vi "Config Reference Point.vi"(8 "error in":errorcluster, 9 "Loss (0 jpF)":dbl min=-99999999.0 max=99999999.0 format="%#_10f", 10 "Capacitance (0 pF)":dbl min=-99999999.0 max=99999999.0 format="%#_10f", 11 "VISA resource name":refnum<visa-resource-name>) -> (0 "error out":errorcluster, 3 "VISA resource name out":refnum<visa-resource-name>)   [LabVIEW 2019, in "Andeen-Hagerling 2700(400 firmware).lvlib"]
doc: "Provides a means for manually entering the capacitance and or loss Reference points."
uses:
  Andeen-Hagerling 2700(400 firmware).lvlib
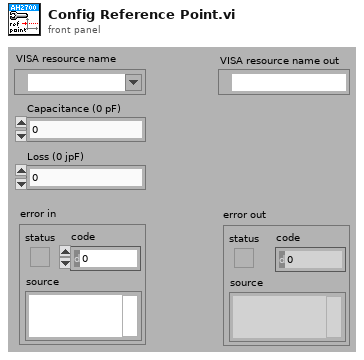
[diagram p1: front panel]
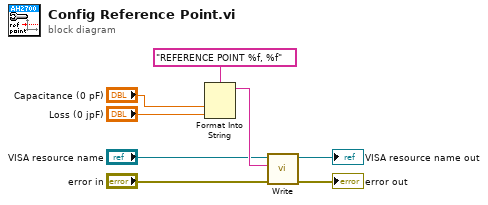
[diagram p0: block diagram]
diagram:
  n1 = Format Into String(format string="REFERENCE POINT %f, %f", "Capacitance (0 pF)", "Loss (0 jpF)") -> (resulting string=w8:string)  [unwired: 2 in, 1 out]
  n2 = call "Write.vi"("error in"="error in", "command"=w8, "VISA resource name"="VISA resource name") -> ("error out"=→"error out":errorcluster, "VISA resource name out"=→"VISA resource name out":refnum<visa-resource-name>)  [unwired: 7 in]
